vi "Test_ReadItem_NotFound_ReturnTypeDefault.vi"(8 "error in (no error)":errorcluster, 11 "TestCase in":refnum<class "TestComposedLookupTable.lvclass">) -> (0 "error out":errorcluster, 3 "TestCase out":refnum<class "TestComposedLookupTable.lvclass">)   [LabVIEW 2017, in "TestComposedLookupTable.lvclass"]
uses:
  TestComposedLookupTable.lvclass
  Source/LookupTable/LookupTable.lvclass/LookupTable.ctl
  01d6e16f-4164-4d05-a2e0-2f61dda92b48.vi
  Source/LookupTable/Read Table Reference.vi
  01d6e16f-4164-4d05-a2e0-2f61dda92b48.vi/1721e68d-11b4-433a-8d9d-ac3e9b4b65d0.vi
  Source/LookupTable/LookupTable.lvclass
panel:
  out "Value":i32
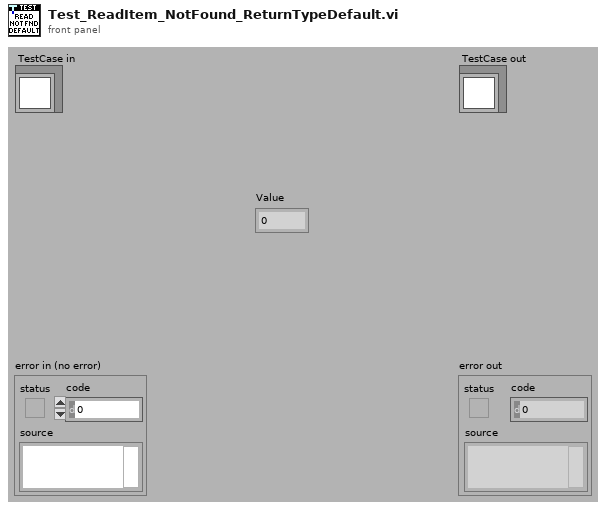
[diagram p1: front panel]
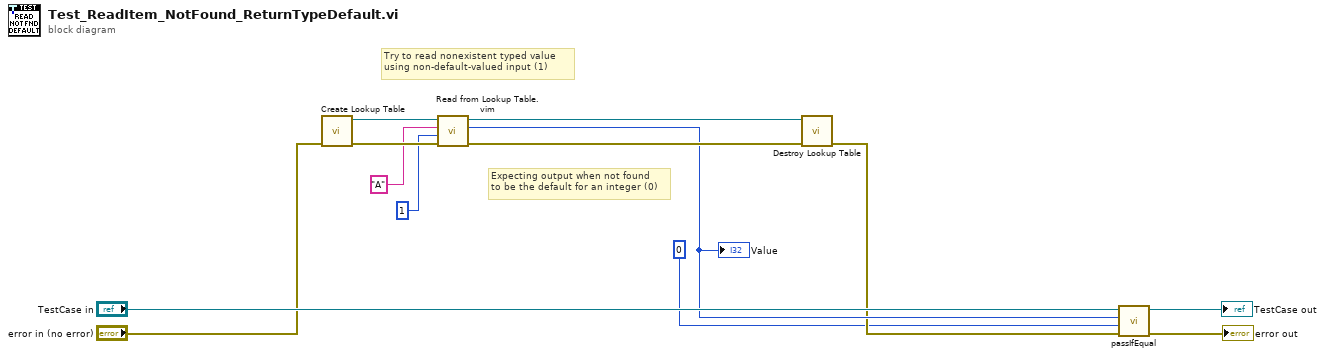
[diagram p0: block diagram]
diagram:
  # "Expecting output when not found\nto be the default for an integer (0)"
  # "Try to read nonexistent typed value\nusing non-default-valued input (1)"
  n1 = call "Create Lookup Table.vi"("error in (no error)"="error in (no error)") -> ("error out"=w12:errorcluster, "LookupTable Reference"=w2:refnum<data-value>)  [unwired: 9 in]
  n2 = call "Read from Lookup Table.vim"("error in (no error)"=w12, "Type"=1, "Item Name"="A", "LookupTable Reference"=w2) -> ("error out"=w13:errorcluster, "Value"=w8:i32, "LookupTable Reference Out"=w5:refnum<data-value>)  [unwired: 4 in, 1 out]
  "Value" <- w8
  n3 = call "Destroy Lookup Table.vi"("error in (no error)"=w13, "LookupTable Reference"=w5) -> ("error out"=w4:errorcluster)  [unwired: 9 in]
  n4 = call-dynamic "passIfEqual.vi"("error in (no error)"=w4, "y"=0, "x"=w8, "TestCase in"="TestCase in") -> ("error out"=→"error out":errorcluster, "TestCase out"=→"TestCase out":refnum<class "TestComposedLookupTable.lvclass">)  [unwired: 6 in]
